vi "Write File.vi"(7 "Channel Direction":string, 8 "error in (no error)":errorcluster, 10 "Channels":refnum<class "Channel.lvclass">[](array[class]), 11 "ConfigFile in":refnum<class "ConfigFile.lvclass">) -> (0 "error out":errorcluster, 3 "ConfigFile out":refnum<class "ConfigFile.lvclass">)   [LabVIEW 2020, in "ImportExport.lvlib"]
uses:
  ImportExport.lvlib
  ConfigFile/ConfigFile.lvclass
  built/windows/Channel.lvlibp/Channel.lvclass
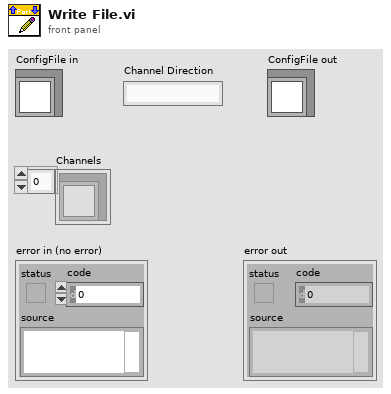
[diagram p1: front panel]
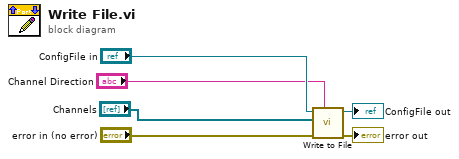
[diagram p0: block diagram]
diagram:
  n1 = call-dynamic "Write to File.vi"("Channel Direction"="Channel Direction", "error in (no error)"="error in (no error)", "Channels"="Channels", "ConfigFile in"="ConfigFile in") -> ("error out"=→"error out":errorcluster, "ConfigFile out"=→"ConfigFile out":refnum<class "ConfigFile.lvclass">)  [unwired: 6 in]
